vi "SetPicture.vi"(6 "TransparentColor":fxp<+,3,3>, 8 "error in (no error)":errorcluster, 9 "ImagePath":path, 10 "SpriteIndex":u8, 11 "SpriteHandler in":refnum<class "SpriteHandler.lvclass">) -> (0 "error out":errorcluster, 3 "SpriteHandler out":refnum<class "SpriteHandler.lvclass">)   [LabVIEW 2019, in "RT_Game.lvlib" / "SpriteHandler.lvclass"]
uses:
  SpriteHandler.lvclass
  SpriteHandler.lvclass/SpriteHandler.ctl
  GameObject/GameObject.lvclass/GameObject.ctl
  GameObject/Write IsActive.vi
  RT_Sprite/RT_Sprite.lvclass
  C:/Users/FreshBob/Dropbox/VIs/myRIO_GameConsole/RT/RT_Game/GameObject/GameObject.lvclass
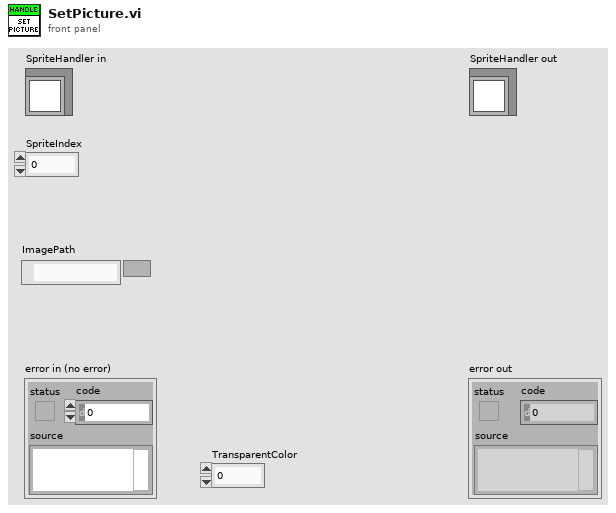
[diagram p1: front panel]
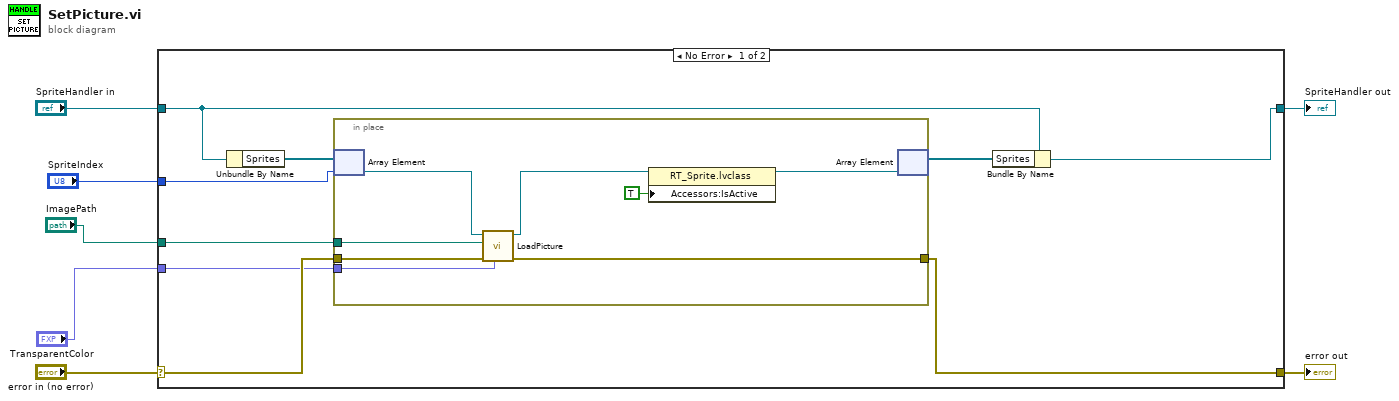
[diagram p0: block diagram]
diagram:
  n1 = case shown="No Error" "error in (no error)" {
    selector: "error in (no error)" -> [w11 w26]
    tunnel: [w10 w26] -> w6
    tunnel: [w13 w25] -> w4
    tunnel: "SpriteHandler in" -> [w16 w25]
    tunnel: "SpriteIndex" -> [w14 _]
    tunnel: "ImagePath" -> [w9 _]
    tunnel: "TransparentColor" -> [w8 _]
    frame No Error {
      n2 = Unbundle By Name(w16) -> ("Sprites"=w15:refnum<class "RT_Sprite.lvclass">[])
      n3 = in-place {
        in-place-border: w11 -> [w24]
        in-place-border: [w23] -> w10
        in-place-border: w9 -> [w20]
        in-place-border: w8 -> [w19]
        n4 = in-place-array #1(w15, w14) -> (w22:refnum<class "RT_Sprite.lvclass">)
        n5 = call "LoadPicture.vi"("Transparent Color"=w19, "error in (no error)"=w24, "Picture Path"=w20, "RT_Sprite in"=w22) -> ("error out"=w23:errorcluster, "RT_Sprite out"=w21:refnum<class "RT_Sprite.lvclass">)  [unwired: 6 in]
        n6 = property class="RT_Sprite.lvclass"(reference=w21, "Accessors:IsActive"=TRUE ("IsActive")) -> (reference out=w18:refnum<class "RT_Sprite.lvclass">)  [unwired: 1 in, 1 out]
        n7 = in-place-array #1(w18) -> (w12:refnum<class "RT_Sprite.lvclass">[])  [unwired: 1 out]
      }
      n8 = Bundle By Name(cluster=w16, "Sprites"=w12) -> (w13:refnum<class "SpriteHandler.lvclass">)
    }
    frame Error {
    }
  }
  "error out" <- w6
  "SpriteHandler out" <- w4
